vi "FTW-ERR-StatusException.vi"(1 "error to check":errorcluster) -> (0 "Exception":T1)   [LabVIEW 2015]
uses:
  FTW-ERR-ExceptionType.ctl
panel:
  # "Inputs"
  # "Outputs"
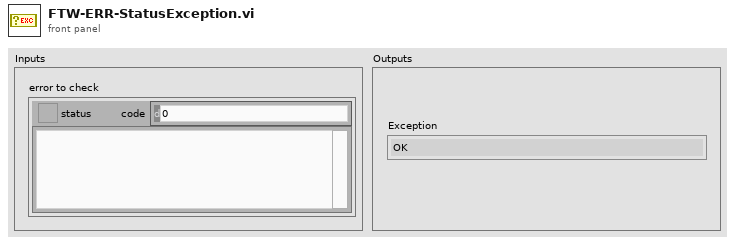
[diagram p1: front panel]
types:
  T1 = typedef "FTW-ERR-ExceptionType.ctl" = enum16{"OK", "Info", "Warning", "Error"}
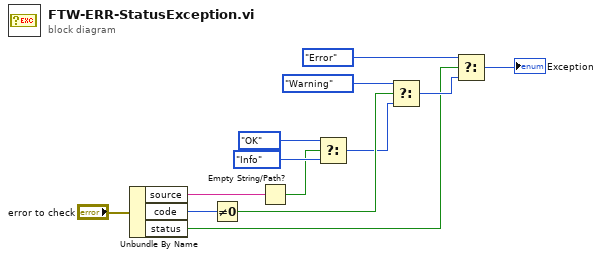
[diagram p0: block diagram]
diagram:
  n1 = Unbundle By Name("error to check") -> ("source"=w5:string, "code"=w13:i32, "status"=w6:bool)
  n2 = Not Equal To 0?(x=w13) -> (x != 0?=w11:bool)
  n3 = Empty String/Path?(string/path=w5) -> (empty?=w2:bool)
  n4 = Select(t=FTW-ERR-ExceptionType."OK" ("Exception"), s=w2, f=FTW-ERR-ExceptionType."Info" ("Exception")) -> (s? t:f=w1:T1)
  n5 = Select(t=FTW-ERR-ExceptionType."Warning" ("Exception"), s=w11, f=w1) -> (s? t:f=w10:T1)
  n6 = Select(t=FTW-ERR-ExceptionType."Error" ("Exception"), s=w6, f=w10) -> (s? t:f=→"Exception":T1)
